vi "Disabled.vi"(7 "Robot Mode":T2, 10 "Match Info":T1={"Autonomous Elapsed Seconds"=0.0, "TeleOp Elapsed Seconds"=0.0, "Disabled Elapsed Seconds"=0.0, "Visited Autonomous"=FALSE, "Visited TeleOp"=FALSE, "Visited Disabled"=FALSE, "Autonomous Settings"={"Autonomous Style"=enum."Independent", "VI Refnum"=refnum}}, 11 "Call Context":T3) -> ()   [LabVIEW 2011]
doc: "This VI is called each time a disabled packet is received from the DS. It is often used to prepare for the next robot mode, to calibrate sensors, etc."
uses:
  <vilib>/Rock Robotics/WPI/DriverStation/WPI_DriverStationDerivedRobotMode.ctl
  <vilib>/Rock Robotics/WPI/DriverStation/WPI_DriverStationRobotMode.ctl
  <vilib>/Rock Robotics/WPI/DriverStation/WPI_DriverStationMatch Info.ctl
  Robot Global Data.vi
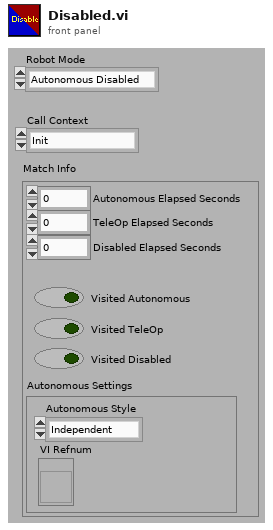
[diagram p1: front panel]
types:
  T1 = typedef "WPI_DriverStationMatch Info.ctl" = cluster{"Autonomous Elapsed Seconds":dbl, "TeleOp Elapsed Seconds":dbl, "Disabled Elapsed Seconds":dbl, "Visited Autonomous":bool, "Visited TeleOp":bool, "Visited Disabled":bool, "Autonomous Settings":cluster{"Autonomous Style":enum16{"Iterative", "Independent"}, "VI Refnum":refnum<vi>}}
  T2 = typedef "WPI_DriverStationRobotMode.ctl" = enum16{"Autonomous Disabled", "Autonomous Enabled", "Teleop Disabled", "Teleop Enabled", "Timeout", "Finish"}
  T3 = typedef "WPI_DriverStationDerivedRobotMode.ctl" = enum16{"Init", "Execute", "Stop"}
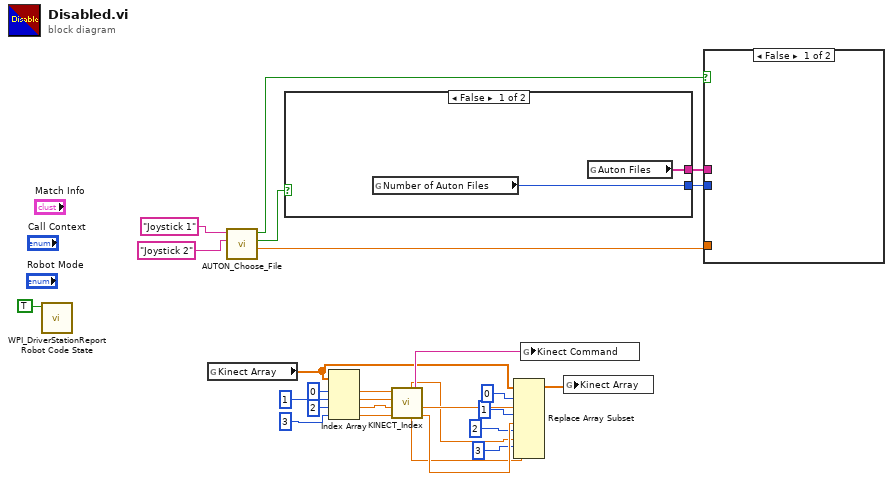
[diagram p0: block diagram]
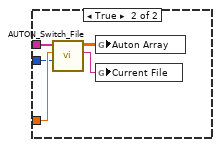
[diagram p2: hidden frame]
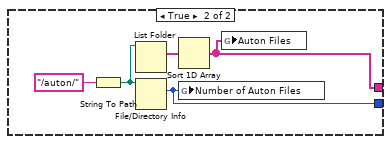
[diagram p3: hidden frame]
diagram:
  n1 = call <vilib>:"WPI_DriverStationReport Robot Code State.vi"("Disabled"=TRUE ("Autonomous")) -> ()  [unwired: 10 in, 1 out]
  n2 = global read "Robot Global Data.vi" "Kinect Array"() -> (w17:dbl[])
  n3 = call "AUTON_Choose_File.vi"("Joystick 2 Refnum"="Joystick 2" ("refnum name"), "Joystick 1 Refnum"="Joystick 1" ("refnum name")) -> ("Auton File"=w1:dbl, "Refresh"=w3:bool, "Allow Change"=w2:bool)  [unwired: 7 in]
  n4 = case shown="False" w3 {
    tunnel: [w28 w31] -> w6
    tunnel: [w29 w30] -> w7
    frame False {
      n5 = global read "Robot Global Data.vi" "Number of Auton Files"() -> (w28:i64)
      n6 = global read "Robot Global Data.vi" "Auton Files"() -> (w29:string[])
    }
    frame True {
      n7 = String To Path(string="/auton/") -> (path=w33:path)
      n8 = List Folder(path=w33) -> (filenames=w32:string[])  [unwired: 1 in, 5 out]
      n9 = File/Directory Info(path=w33) -> (size=w31:i64)  [unwired: 1 in, 6 out]
      n10 = Sort 1D Array(array=w32) -> (sorted array=w30:string[])
      n11 = global write "Robot Global Data.vi" "Number of Auton Files"(w31) -> ()
      n12 = global write "Robot Global Data.vi" "Auton Files"(w30) -> ()
    }
  }
  n13 = Index Array(array=w17, index #1=0 ("index"), index #2=1 ("index"), index #3=2 ("index"), index #4=3 ("index")) -> (element #1=w21:dbl, element #2=w20:dbl, element #3=w19:dbl, element #4=w18:dbl)
  n14 = call "KINECT_Index.vi"("Arm Drive Min in (Reverse)"=w18, "Arm Drive Max in (Forward)"=w19, "Z Wrist Left"=w20, "Z Wrist Right"=w21) -> ("Z Wrist Left"=w13:sgl, "Z Wrist Right"=w15:sgl, "Kinect Command"=w26:string, "Arm Drive Min out (Reverse)"=w9:dbl, "Arm Drive Max out (Forward)"=w10:dbl)  [unwired: 3 in]
  n15 = Replace Array Subset(array=w17, new element #1=w15, index #1=0 ("index"), new element #2=w13, index #2=1 ("index"), new element #3=w10, index #3=2 ("index"), new element #4=w9, index #4=3 ("index")) -> (w8:dbl[])
  n16 = global write "Robot Global Data.vi" "Kinect Command"(w26) -> ()
  n17 = global write "Robot Global Data.vi" "Kinect Array"(w8) -> ()
  n18 = case shown="False" w2 {
    tunnel: w1 -> [_ w37]
    tunnel: w7 -> [_ w36]
    tunnel: w6 -> [_ w35]
    frame False {
    }
    frame True {
      n19 = call "AUTON_Switch_File.vi"("Number of Auton Files"=w35, "Auton File"=w37, "Auton Files"=w36) -> ("Current File"=w38:string, "Auton Array"=w39:dbl[][])  [unwired: 7 in]
      n20 = global write "Robot Global Data.vi" "Auton Array"(w39) -> ()
      n21 = global write "Robot Global Data.vi" "Current File"(w38) -> ()
    }
  }
